vi "camera attribute.vi"(10 "ParameterIn":string, 11 "CamName":string) -> (2 "Btn_Cancel 2":bool, 3 "DataOut":string)   [LabVIEW 2019]
uses:
  Ctrl/VisionProcessName.ctl
  Controls/CameraAttribute.ctl
  <vilib>/Utility/miscctls.llb/LVPointTypeDef.ctl
  Controls/Process_Setting.ctl
  032adceb-56a2-4fae-8e21-1bd23329ef5e.vi
  f0b30054-bd93-4fdd-8b7e-7129c6357697.vi
  6001ebed-b65a-49e9-9159-11edffe4d8f3.vi
  a7ab80fa-e7a2-4b62-8649-8d751b667496.vi
  <vilib>/JDP Science/JSONtext/JSON text to Variant.vi
  <vilib>/JDP Science/JSONtext/Variant to JSON Text.vi
  <resource>/objmgr/imaqdx.rc
panel:
  out "CamIndex":i32
  out "CamAttribute":T1
  in  "Enum_PreProcess":T2
  in  "Tab Control":enum32{"Page 1", "Page 2"}(tab)
  in  "Gain":dbl
  in  "Exposure":dbl
  out "Image":T3(plugin-control)
  in  "AutoExposure":enum16{"Off", "Once", "Continuous"}(ring)
  in  "AutoGain":enum16{"Off", "Once", "Continuous"}(ring)
  in  "Btn_Set":bool
  in  "Btn_Cancel":bool
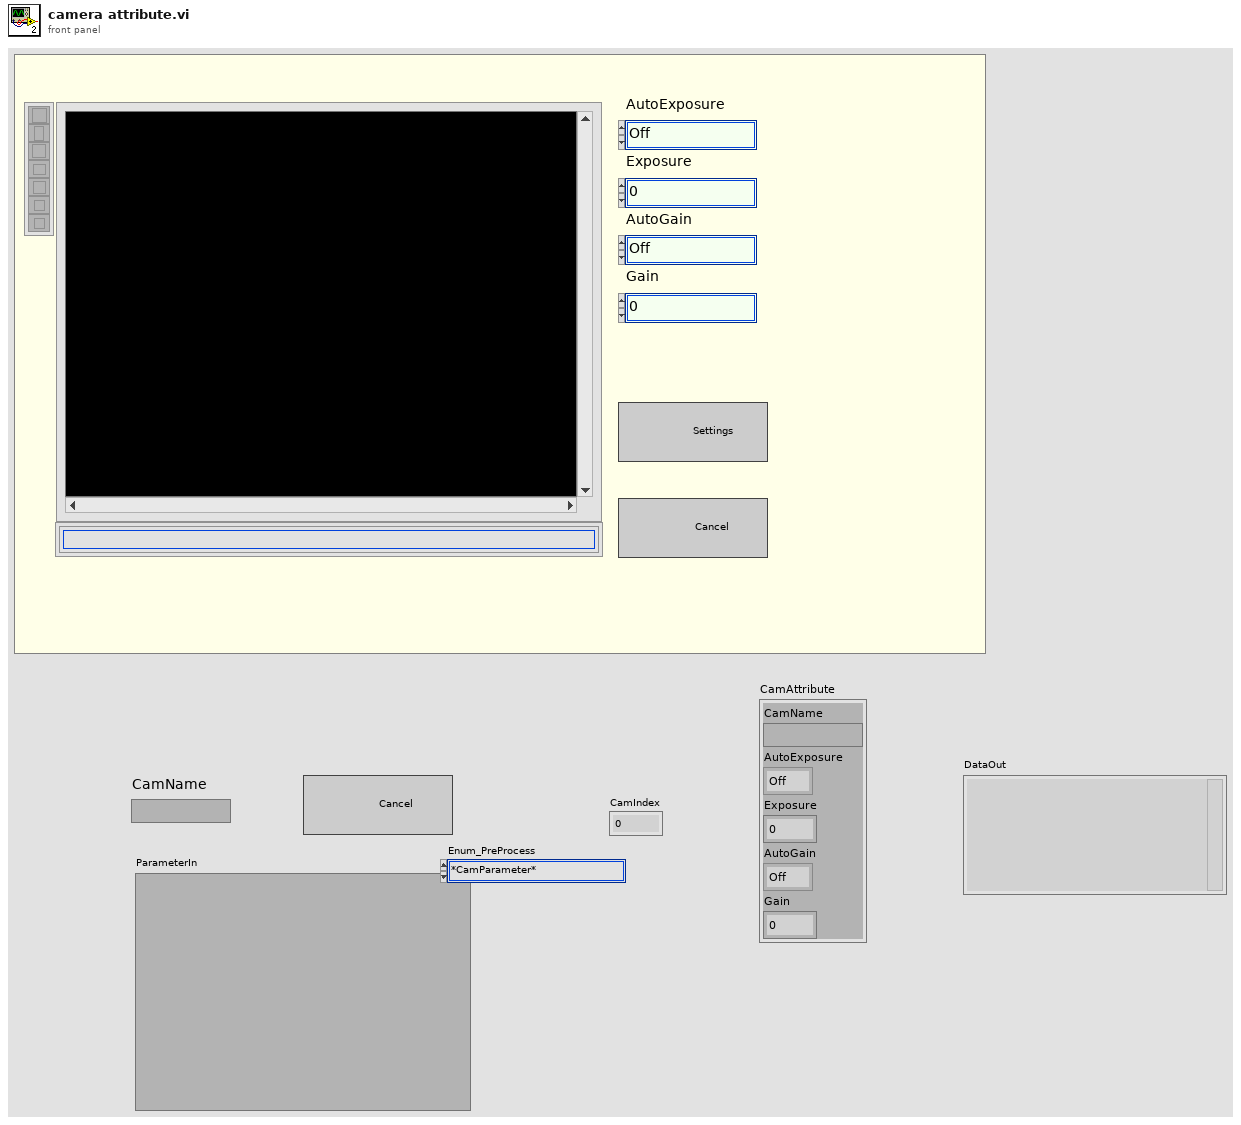
[diagram p1: front panel]
types:
  T1 = typedef "CameraAttribute.ctl" = cluster{"CamName":string, "AutoExposure":enum16{"Off", "Once", "Continuous"}, "Exposure":dbl, "AutoGain":enum16{"Off", "Once", "Continuous"}, "Gain":dbl}
  T2 = typedef "VisionProcessName.ctl" = enum16{"*CamParameter*", "CamAttributes", "*Preprocess*", "CG_Brightness", "C_Plane Extraction", "C_Threshold", "G_Lookup Table", "G_Threshold"}
  T3 = typedef "IMAQ Image.ctl" = refnum<image>
  T4 = typedef "LVPointTypeDef.ctl" = cluster{"Horizontal":i16, "Vertical":i16}
  T5 = enum16{"Init", "Grab", "Get All", "Close", "Set Camera"}
  T6 = typedef "Process_Setting.ctl" = cluster{"Enum_PreProcess":T2, "Parameter":string}
  T7 = typedef "IMAQdx.ctl" = refnum<k21>
  T8 = cluster{"CamName":string, "AutoExposure":enum16{"Off", "Once", "Continuous"}, "Exposure":dbl, "AutoGain":enum16{"Off", "Once", "Continuous"}, "Gain":dbl}
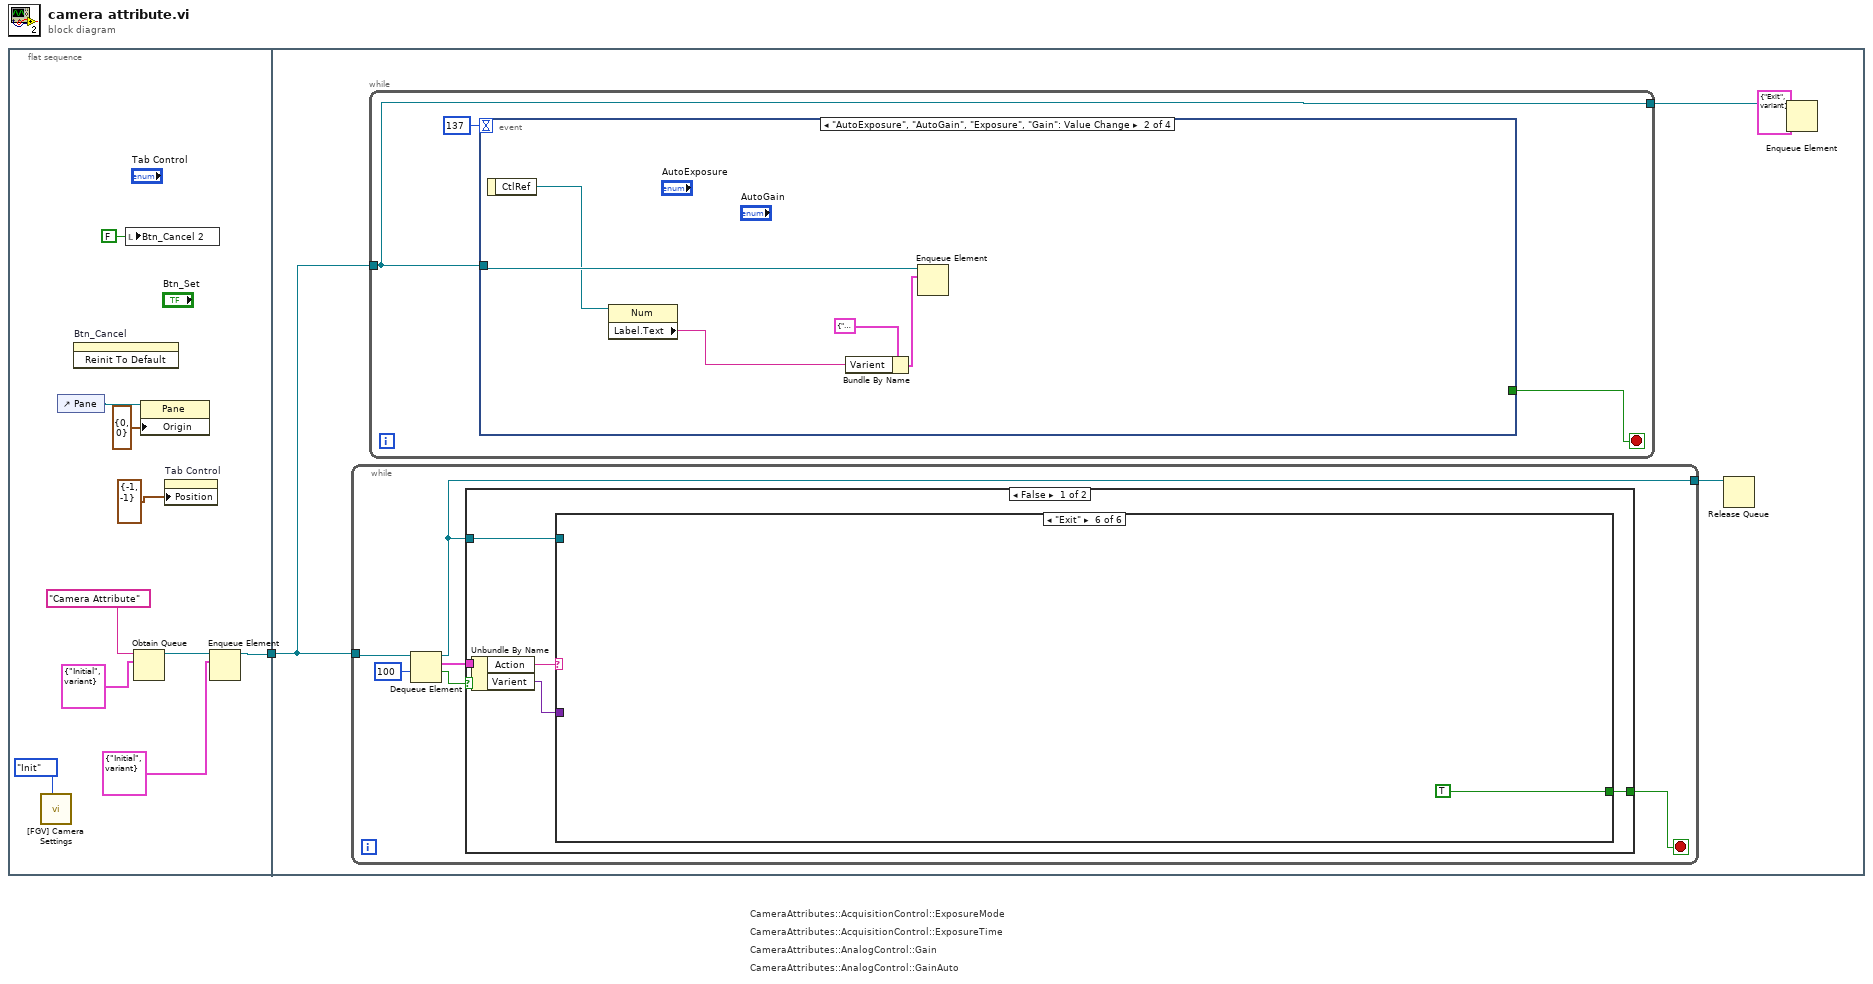
[diagram p0: block diagram]
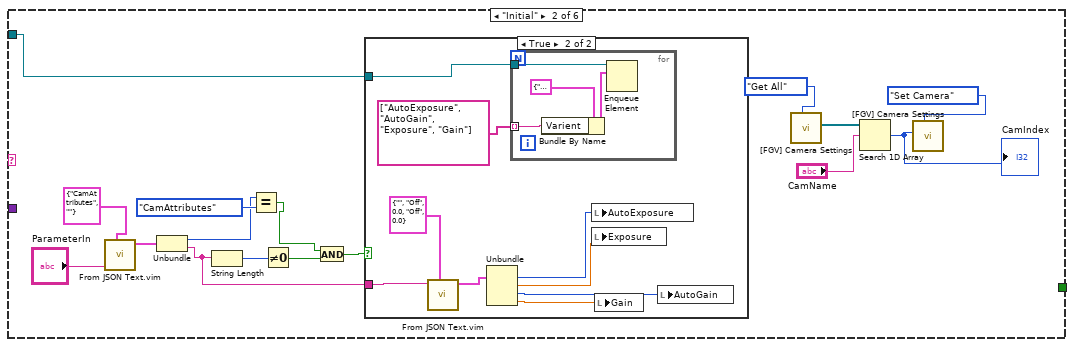
[diagram p3: hidden frame]
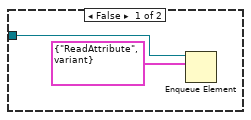
[diagram p4: hidden frame]
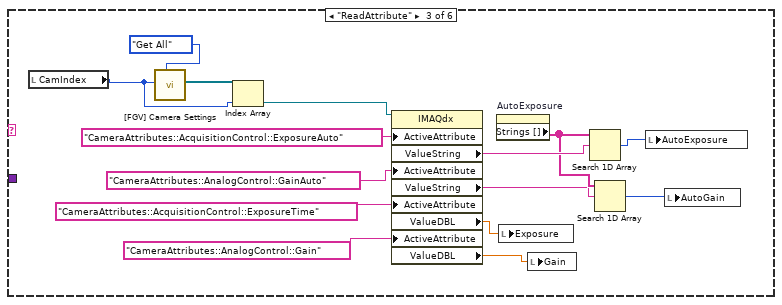
[diagram p5: hidden frame]
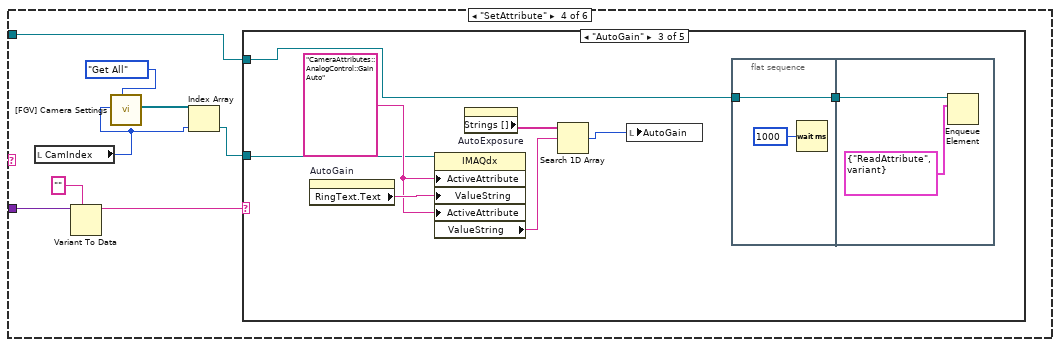
[diagram p6: hidden frame]
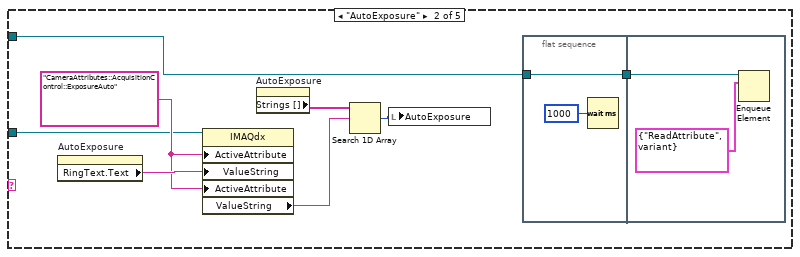
[diagram p8: hidden frame]
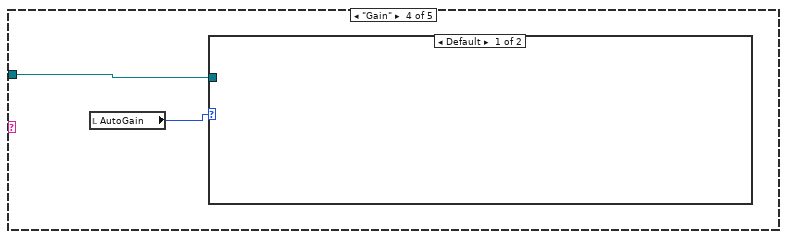
[diagram p9: hidden frame]
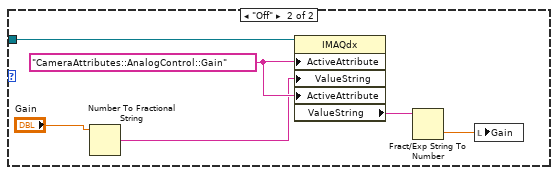
[diagram p10: hidden frame]
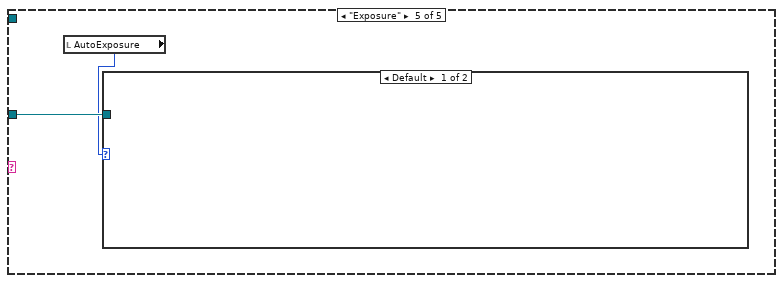
[diagram p11: hidden frame]
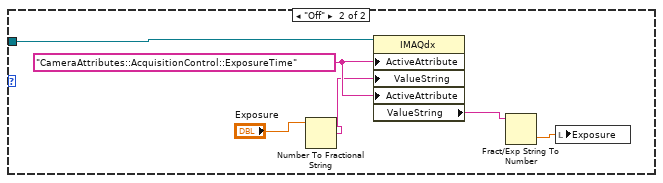
[diagram p12: hidden frame]
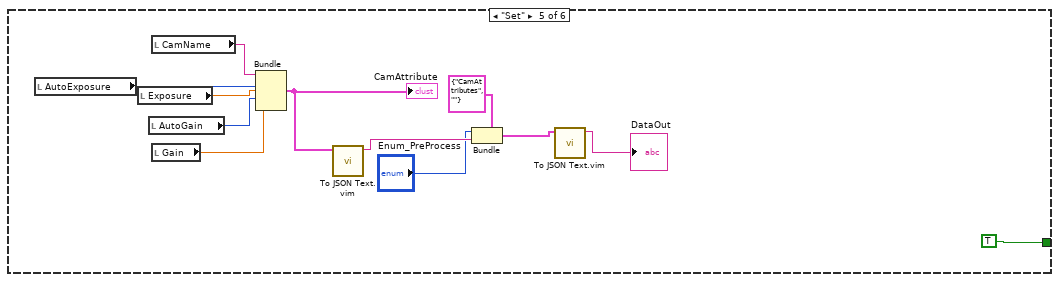
[diagram p13: hidden frame]
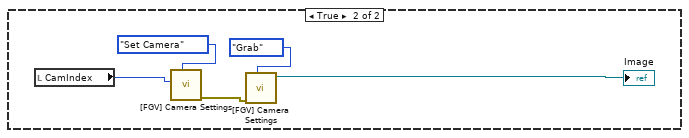
[diagram p14: hidden frame]
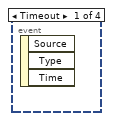
[diagram p15: hidden frame]
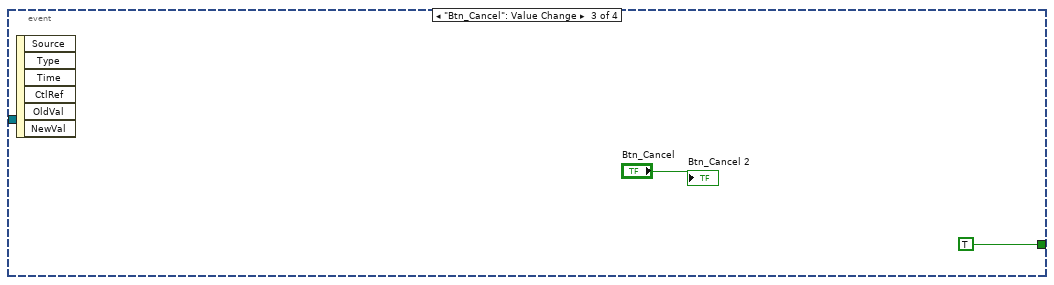
[diagram p16: hidden frame]
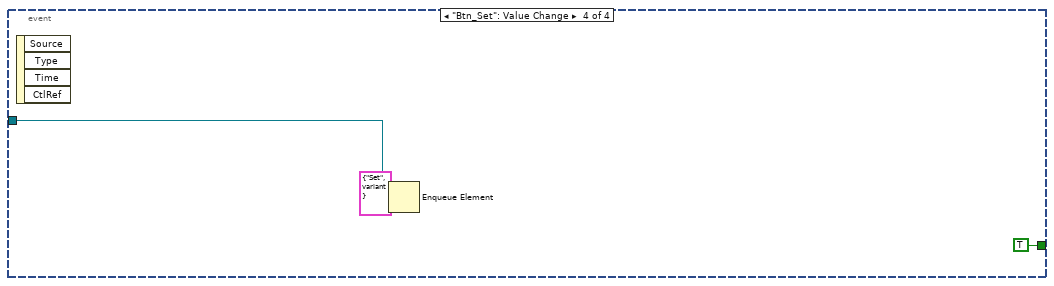
[diagram p17: hidden frame]
diagram:
  # "CameraAttributes::AnalogControl::GainAuto"
  # "CameraAttributes::AnalogControl::Gain"
  # "CameraAttributes::AcquisitionControl::ExposureMode"
  # "CameraAttributes::AcquisitionControl::ExposureTime"
  n1 = flat-sequence {
    tunnel: [w7] -> w1
    tunnel: w1 -> [w15]
    frame #0 {
      n2 = call "[FGV] Camera Settings.vi"("Action"=T5."Init") -> ()  [unwired: 8 in, 3 out]
      n3 = control-ref of="Pane"() -> (w5:refnum<vi>)
      n4 = invoke on="Btn_Cancel" class="Bool (strict)" method="Reinit To Default"() -> ()  [unwired: 3 in, 3 out]
      n5 = local write "Btn_Cancel 2"(FALSE ("Btn_Cancel 2")) -> ()
      n6 = Obtain Queue(name (unnamed)="Camera Attribute", element data type=cluster{"Action":string, "Varient":variant} {"Action"="Initial", "Varient"=variant} ("element")) -> (queue out=w8:refnum<queue>)  [unwired: 3 in, 2 out]
      n7 = property class="Pane"(reference=w5, "Origin"=T4 {"Horizontal"=0, "Vertical"=0}) -> ()  [unwired: 1 in, 2 out]
      n8 = property on="Tab Control" class="TabCtl (strict)"("Position"=T4 {"Horizontal"=-1, "Vertical"=-1} ("Origin")) -> ()  [unwired: 2 in, 2 out]
      n9 = Enqueue Element(queue=w8, element=cluster{"Action":string, "Varient":variant} {"Action"="Initial", "Varient"=variant}) -> (queue out=w7:refnum<queue>)  [unwired: 2 in, 2 out]
    }
    frame #1 {
      n10 = while {
        tunnel: w15 -> [w21]
        tunnel: [w16] -> w12
        stop <- w17 stop-if-true
        n11 = Dequeue Element(queue=w21, timeout in ms (-1)=100) -> (queue out=w16:refnum<queue>, element=w20:cluster{"Action":string, "Varient":variant}, timed out?=w18:bool)  [unwired: 1 in, 1 out]
        n12 = case shown="False" w18 {
          tunnel: w20 -> [w26 _]
          tunnel: [w24 _] -> w17
          tunnel: w16 -> [w22 _]
          frame False {
            n13 = Unbundle By Name(w26) -> ("Action"=w25:string, "Varient"=w23:variant)
            n14 = case shown="\"Exit\"" w25 {
              tunnel: [_ _ _ _ TRUE TRUE] -> w24
              tunnel: w23 -> [_ _ _ w80 _ _]
              tunnel: w22 -> [_ w33 _ w74 _ _]
              frame "False", Default {
              }
              frame "Initial" {
                n15 = call "From JSON Text.vim"("Data Type and Default Value"=T6 {"Enum_PreProcess"=enum."CamAttributes", "Parameter"=""} ("ProcessSetting"), "JSON"="ParameterIn") -> ("Data out"=w40:T6)  [unwired: 8 in, 1 out]
                n16 = Unbundle(w40) -> ("Enum_PreProcess"=w38:T2, "Parameter"=w32:string)
                n17 = String Length(string=w32) -> (length=w37:i32)
                n18 = Equal?(x=w38, y=VisionProcessName."CamAttributes") -> (x = y?=w35:bool)
                n19 = Not Equal To 0?(x=w37) -> (x != 0?=w36:bool)
                n20 = And(x=w35, y=w36) -> (x .and. y?=w34:bool)
                n21 = case shown="True" w34 {
                  tunnel: w33 -> [w44 w46]
                  tunnel: w32 -> [_ w53]
                  frame False {
                    n22 = Enqueue Element(queue=w44, element=cluster{"Action":string, "Varient":variant} {"Action"="ReadAttribute", "Varient"=variant}) -> ()  [unwired: 2 in, 3 out]
                  }
                  frame True {
                    n23 = call "From JSON Text.vim"("Data Type and Default Value"=T1 {"CamName"="", "AutoExposure"=enum."Off", "Exposure"=0.0, "AutoGain"=enum."Off", "Gain"=0.0} ("CamAttribute"), "JSON"=w53) -> ("Data out"=w51:T1)  [unwired: 8 in, 1 out]
                    n24 = Unbundle(w51) -> ("AutoExposure"=w47:enum16{"Off", "Once", "Continuous"}, "Exposure"=w48:dbl, "AutoGain"=w49:enum16{"Off", "Once", "Continuous"}, "Gain"=w50:dbl)  [unwired: 1 out]
                    n25 = for {
                      tunnel: w46 -> [w55]
                      tunnel: string[] ["AutoExposure", "AutoGain", "Exposure", "Gain"] -> [w54] mode=indexing
                      n26 = Bundle By Name(cluster=cluster{"Action":string, "Varient":variant} {"Action"="SetAttribute", "Varient"=variant} ("element"), "Varient"=w54) -> (w57:cluster{"Action":string, "Varient":variant})
                      n27 = Enqueue Element(queue=w55, element=w57) -> ()  [unwired: 2 in, 3 out]
                    }
                    n28 = local write "AutoExposure"(w47) -> ()
                    n29 = local write "Exposure"(w48) -> ()
                    n30 = local write "Gain"(w50) -> ()
                    n31 = local write "AutoGain"(w49) -> ()
                  }
                }
                n32 = call "[FGV] Camera Settings.vi"("Action"=T5."Get All") -> ("Camera Interface Name"=w31:T7[])  [unwired: 8 in, 2 out]
                n33 = Search 1D Array(1D array=w31, element="CamName") -> (index of element=w30:i32)  [unwired: 1 in]
                "CamIndex" <- w30
                n34 = call "[FGV] Camera Settings.vi"("Action"=T5."Set Camera", "Value"=w30) -> ()  [unwired: 7 in, 3 out]
              }
              frame "ReadAttribute" {
                n35 = local read "CamIndex"() -> (w58:i32)
                n36 = call "[FGV] Camera Settings.vi"("Action"=T5."Get All", "Value"=w58) -> ("Camera Interface Name"=w71:T7[])  [unwired: 7 in, 2 out]
                n37 = Index Array(array=w71, index=w58) -> (element=w70:T7)
                n38 = property class="IMAQdx"(reference=w70, "ActiveAttribute"="CameraAttributes::AcquisitionControl::ExposureAuto", "ActiveAttribute"="CameraAttributes::AnalogControl::GainAuto", "ActiveAttribute"="CameraAttributes::AcquisitionControl::ExposureTime", "ActiveAttribute"="CameraAttributes::AnalogControl::Gain") -> ("ValueString"=w68:string, "ValueString"=w65:string, "ValueDBL"=w59:dbl, "ValueDBL"=w60:dbl)  [unwired: 1 in, 2 out]
                n39 = property on="AutoExposure" class="Enum (strict)"() -> ("Strings []"=w66:string[])  [unwired: 2 in, 2 out]
                n40 = local write "Exposure"(w59) -> ()
                n41 = local write "Gain"(w60) -> ()
                n42 = Search 1D Array(1D array=w66, element=w68) -> (index of element=w67:i32)  [unwired: 1 in]
                n43 = Search 1D Array(1D array=w66, element=w65) -> (index of element=w64:i32)  [unwired: 1 in]
                n44 = local write "AutoExposure"(w67) -> ()
                n45 = local write "AutoGain"(w64) -> ()
              }
              frame "SetAttribute" {
                n46 = local read "CamIndex"() -> (w73:i32)
                n47 = Variant To Data(type="", Variant=w80) -> (data=w78:string)  [unwired: 1 in, 1 out]
                n48 = call "[FGV] Camera Settings.vi"("Action"=T5."Get All", "Value"=w73) -> ("Camera Interface Name"=w77:T7[])  [unwired: 7 in, 2 out]
                n49 = Index Array(array=w77, index=w73) -> (element=w75:T7)
                n50 = case shown="\"AutoGain\"" w78 {
                  tunnel: w75 -> [_ w83 w95 w106 w114]
                  tunnel: w74 -> [_ w82 w93 _ _]
                  frame "False", Default {
                  }
                  frame "AutoExposure" {
                    w84 = "CameraAttributes::AcquisitionControl::ExposureAuto" ("ActiveAttribute")
                    n51 = property on="AutoExposure" class="Enum (strict)"() -> ("RingText.Text"=w85:string)  [unwired: 2 in, 2 out]
                    n52 = property class="IMAQdx"(reference=w83, "ActiveAttribute"=w84, "ValueString"=w85, "ActiveAttribute"=w84) -> ("ValueString"=w88:string)  [unwired: 1 in, 2 out]
                    n53 = property on="AutoExposure" class="Enum (strict)"() -> ("Strings []"=w86:string[])  [unwired: 2 in, 2 out]
                    n54 = Search 1D Array(1D array=w86, element=w88) -> (index of element=w87:i32)  [unwired: 1 in]
                    n55 = local write "AutoExposure"(w87) -> ()
                    n56 = flat-sequence {
                      tunnel: w82 -> [w90]
                      tunnel: [w90] -> w81
                      tunnel: w81 -> [w91]
                      frame #0 {
                        n57 = Wait (ms)(milliseconds to wait=u32 1000) -> ()  [unwired: 1 out]
                      }
                      frame #1 {
                        n58 = Enqueue Element(queue=w91, element=cluster{"Action":string, "Varient":variant} {"Action"="ReadAttribute", "Varient"=variant}) -> ()  [unwired: 2 in, 3 out]
                      }
                    }
                  }
                  frame "AutoGain" {
                    w96 = "CameraAttributes::AnalogControl::GainAuto" ("ActiveAttribute")
                    n59 = property on="AutoGain" class="Enum (strict)"() -> ("RingText.Text"=w97:string)  [unwired: 2 in, 2 out]
                    n60 = property class="IMAQdx"(reference=w95, "ActiveAttribute"=w96, "ValueString"=w97, "ActiveAttribute"=w96) -> ("ValueString"=w100:string)  [unwired: 1 in, 2 out]
                    n61 = property on="AutoExposure" class="Enum (strict)"() -> ("Strings []"=w98:string[])  [unwired: 2 in, 2 out]
                    n62 = Search 1D Array(1D array=w98, element=w100) -> (index of element=w99:i32)  [unwired: 1 in]
                    n63 = local write "AutoGain"(w99) -> ()
                    n64 = flat-sequence {
                      tunnel: w93 -> [w102]
                      tunnel: [w102] -> w94
                      tunnel: w94 -> [w103]
                      frame #0 {
                        n65 = Wait (ms)(milliseconds to wait=u32 1000) -> ()  [unwired: 1 out]
                      }
                      frame #1 {
                        n66 = Enqueue Element(queue=w103, element=cluster{"Action":string, "Varient":variant} {"Action"="ReadAttribute", "Varient"=variant}) -> ()  [unwired: 2 in, 3 out]
                      }
                    }
                  }
                  frame "Gain" {
                    n67 = local read "AutoGain"() -> (w105:enum16{"Off", "Once", "Continuous"})
                    n68 = case shown="Default" w105 {
                      tunnel: w106 -> [_ w111]
                      frame Default {
                      }
                      frame "Off" {
                        w112 = "CameraAttributes::AnalogControl::Gain" ("ActiveAttribute")
                        n69 = Number To Fractional String(number="Gain") -> (F-format string=w109:string)  [unwired: 3 in]
                        n70 = property class="IMAQdx"(reference=w111, "ActiveAttribute"=w112, "ValueString"=w109, "ActiveAttribute"=w112) -> ("ValueString"=w108:string)  [unwired: 1 in, 2 out]
                        n71 = Fract/Exp String To Number(string=w108) -> (number=w107:dbl)  [unwired: 3 in, 1 out]
                        n72 = local write "Gain"(w107) -> ()
                      }
                    }
                  }
                  frame "Exposure" {
                    n73 = local read "AutoExposure"() -> (w113:enum16{"Off", "Once", "Continuous"})
                    n74 = case shown="Default" w113 {
                      tunnel: w114 -> [_ w119]
                      frame Default {
                      }
                      frame "Off" {
                        w120 = "CameraAttributes::AcquisitionControl::ExposureTime" ("ActiveAttribute")
                        n75 = Number To Fractional String(number="Exposure") -> (F-format string=w117:string)  [unwired: 3 in]
                        n76 = property class="IMAQdx"(reference=w119, "ActiveAttribute"=w120, "ValueString"=w117, "ActiveAttribute"=w120) -> ("ValueString"=w116:string)  [unwired: 1 in, 2 out]
                        n77 = Fract/Exp String To Number(string=w116) -> (number=w115:dbl)  [unwired: 3 in, 1 out]
                        n78 = local write "Exposure"(w115) -> ()
                      }
                    }
                  }
                }
              }
              frame "Set" {
                n79 = local read "AutoExposure"() -> (w128:enum16{"Off", "Once", "Continuous"})
                n80 = local read "Exposure"() -> (w129:dbl)
                n81 = local read "AutoGain"() -> (w130:enum16{"Off", "Once", "Continuous"})
                n82 = local read "CamName"() -> (w132:string)
                n83 = local read "Gain"() -> (w131:dbl)
                n84 = Bundle("CamName"=w132, "AutoExposure"=w128, "Exposure"=w129, "AutoGain"=w130, "Gain"=w131) -> (w127:T8)  [unwired: 1 in]
                "CamAttribute" <- w127
                n85 = call "To JSON Text.vim"("Anything"=w127) -> ("<JSON>"=w125:string)  [unwired: 9 in, 1 out]
                n86 = Bundle(cluster=T6 {"Enum_PreProcess"=enum."CamAttributes", "Parameter"=""} ("ProcessSetting"), "Enum_PreProcess"="Enum_PreProcess", "Parameter"=w125) -> (w123:T6)
                n87 = call "To JSON Text.vim"("Anything"=w123) -> ("<JSON>"=→"DataOut":string)  [unwired: 9 in, 1 out]
              }
              frame "Exit" {
              }
            }
          }
          frame True {
            n88 = local read "CamIndex"() -> (w135:i32)
            n89 = call "[FGV] Camera Settings.vi"("Action"=T5."Set Camera", "Value"=w135) -> ("error out"=w136:errorcluster)  [unwired: 7 in, 2 out]
            n90 = call "[FGV] Camera Settings.vi"("Action"=T5."Grab", "error in (no error)"=w136) -> ("Image Out"=→"Image":T3)  [unwired: 7 in, 2 out]
          }
        }
      }
      n91 = while {
        tunnel: [w139] -> w14
        tunnel: w15 -> [w139]
        stop <- w140 stop-if-true
        n92 = event shown="[1] \"AutoExposure\", \"AutoGain\", \"Exposure\", \"Gain\": Value Change" {
          selector: _ -> [_ _ _ _]
          dyn-events: _ -> [_ _ _ _]
          timeout: 137 -> [_ _ _ _]
          tunnel: [_ _ TRUE TRUE] -> w140
          tunnel: w139 -> [_ w146 _ w151]
          event Timeout {
            n93 = event-data() -> ()  [unwired: 1 in, 3 out]
          }
          event "AutoExposure", "AutoGain", "Exposure", "Gain": Value Change {
            n94 = event-data() -> ("CtlRef"=w143:refnum<vi>)  [unwired: 1 in]
            n95 = property class="Num"(reference=w143) -> ("Label.Text"=w142:string)  [unwired: 1 in, 2 out]
            n96 = Bundle By Name(cluster=cluster{"Action":string, "Varient":variant} {"Action"="SetAttribute", "Varient"=variant} ("element"), "Varient"=w142) -> (w144:cluster{"Action":string, "Varient":variant})
            n97 = Enqueue Element(queue=w146, element=w144) -> ()  [unwired: 2 in, 3 out]
          }
          event "Btn_Cancel": Value Change {
            n98 = event-data() -> ()  [unwired: 1 in, 6 out]
            "Btn_Cancel 2" <- "Btn_Cancel"
          }
          event "Btn_Set": Value Change {
            n99 = event-data() -> ()  [unwired: 1 in, 4 out]
            n100 = Enqueue Element(queue=w151, element=cluster{"Action":string, "Varient":variant} {"Action"="Set", "Varient"=variant}) -> ()  [unwired: 2 in, 3 out]
          }
        }
      }
      n101 = Release Queue(queue=w12) -> ()  [unwired: 2 in, 3 out]
      n102 = Enqueue Element(queue=w14, element=cluster{"Action":string, "Varient":variant} {"Action"="Exit", "Varient"=variant}) -> ()  [unwired: 2 in, 3 out]
    }
  }
